vi "Autonomous Independent.vi"   [LabVIEW 2017]
doc: "This VI is called when autonomous begins, and will automatically be terminated when autonomous ends. You can carry out timed or sensor driven robot movement independently without needing to return to the caller."
uses:
  <vilib>/Rock Robotics/WPI/Utilities/WPI_GetSetVariantRefNum.vi
  <vilib>/Rock Robotics/Network Tables/NT Read String.vi
  <vilib>/Rock Robotics/Network Tables/NT Write Numeric Array.vi
panel:
  # "Be sure to right-click and choose Data Operations>>Make Current Value default if you want to save the array values with the VI"
types:
  T1 = typedef "WPI_JoystickDevRef.ctl" = cluster{"Device":T2}
  T2 = typedef "WPI_JoystickDeviceEnum.ctl" = enum16{"USB 0", "USB 1", "USB 2", "USB 3", "USB 4", "USB 5"}
  T3 = typedef "WPI_RobotDriveDevRef.ctl" = cluster{"DevStatus":errorcluster, "Motors[]":T4[], "Square Inputs":bool, "Max Output":dbl}
  T4 = typedef "WPI_MotorControlDeviceRef.ctl" = cluster{"DeviceStatus":errorcluster, "Type":T5, "PWM":cluster{"PWM Channel":T6, "DeadBand":T7}, "CAN":cluster{"Device Number":u8, "SetOutput VI Ref":variant, "GetOutput VI Ref":variant, "Enable VI Ref":variant, "Disable VI Ref":variant, "Data":variant}, "Invert":bool, "DIO PWM":cluster{"PWM \"Enable\" Channel":T6, "DIOChannel":T8, "PWM Rate":dbl}}
  T5 = typedef "WPI_MotorControlType.ctl" = enum16{"PWM", "CAN", "DIO PWM"}
  T6 = typedef "FPGA_DIOPWMChannel.ctl" = enum8{"PWM 0", "PWM 1", "PWM 2", "PWM 3", "PWM 4", "PWM 5", "PWM 6", "PWM 7", "PWM 8", "PWM 9", "PWM MXP 0", "PWM MXP 1", "PWM MXP 2", "PWM MXP 3", "PWM MXP 4", "PWM MXP 5", "PWM MXP 6", "PWM MXP 7", "PWM MXP 8", "PWM MXP 9", "Invalid"}
  T7 = typedef "WPI_PWMDeadband.ctl" = cluster{"Name":string, "maxPositivePwm":i32, "minPositivePwm":i32, "centerPwm":i32, "maxNegativePwm":i32, "minNegativePwm":i32, "angularRange":u16}
  T8 = typedef "FPGA_DIOChannel.ctl" = enum8{"DIO 0", "DIO 1", "DIO 2", "DIO 3", "DIO 4", "DIO 5", "DIO 6", "DIO 7", "DIO 8", "DIO 9", "DIO MXP 0", "DIO MXP 1", "DIO MXP 2", "DIO MXP 3", "DIO MXP 4", "DIO MXP 5", "DIO MXP 6", "DIO MXP 7", "DIO MXP 8", "DIO MXP 9", "DIO MXP 10", "DIO MXP 11", "DIO MXP 12", "DIO MXP 13", "DIO MXP 14", "DIO MXP 15", "SPI Port CS1", "SPI Port CS2", "SPI Port CS3", "SPI Port MISO", "SPI Port MOSI", "Invalid"}
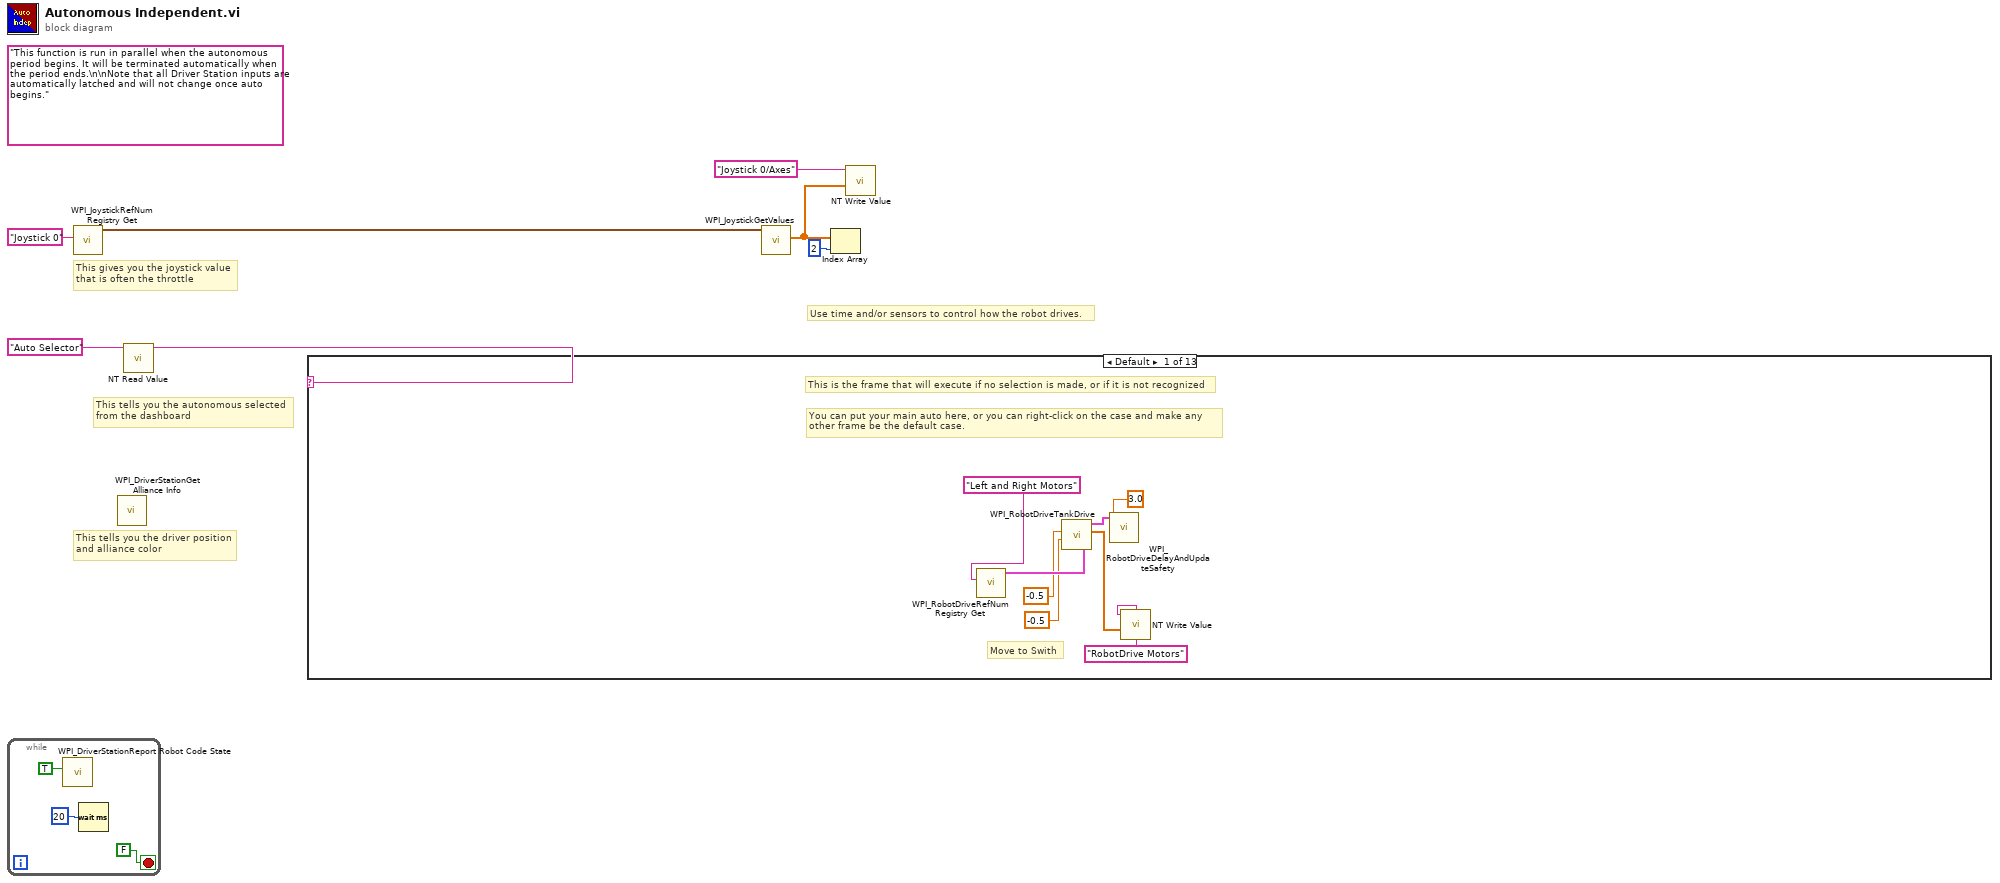
[diagram p0: block diagram]
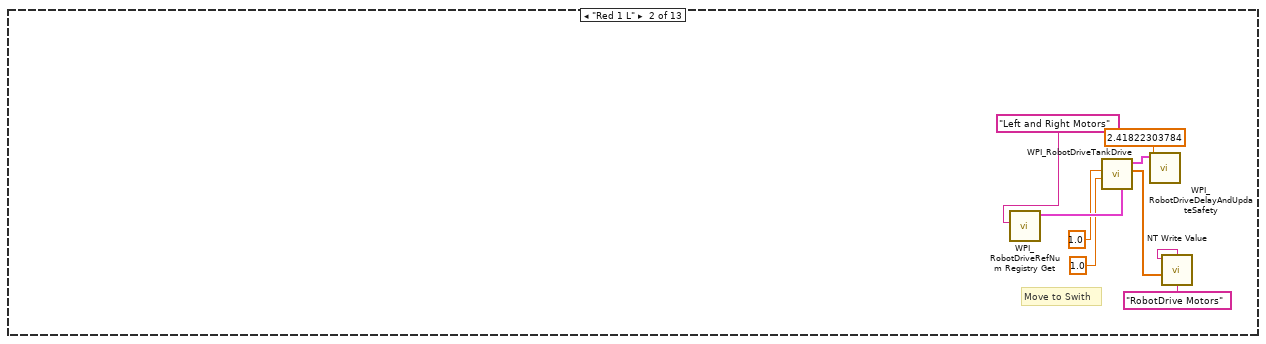
[diagram p2: hidden frame]
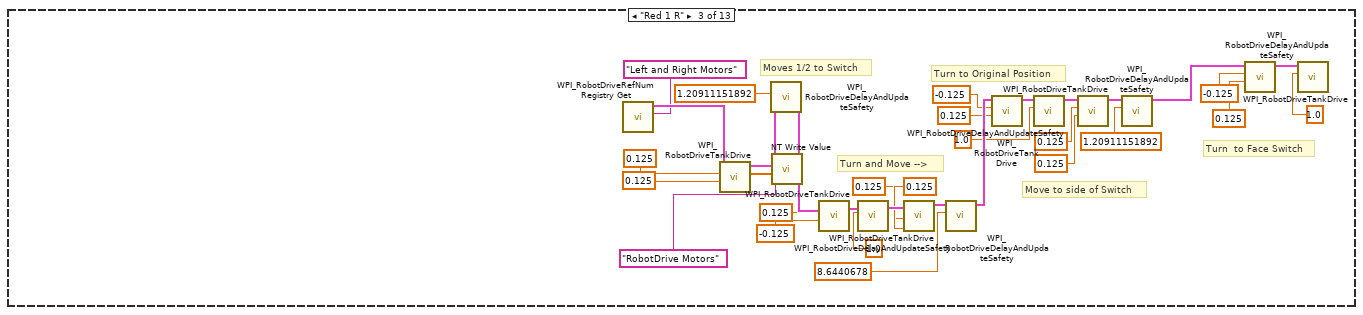
[diagram p3: hidden frame]
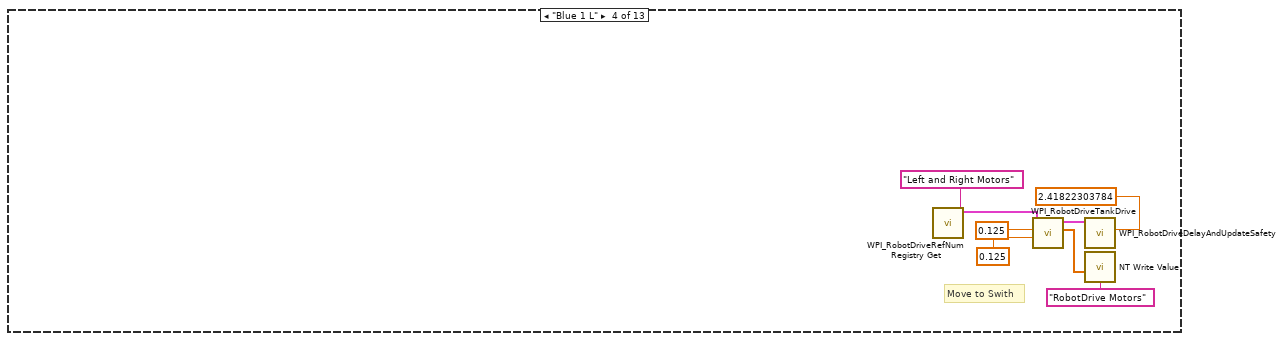
[diagram p4: hidden frame]
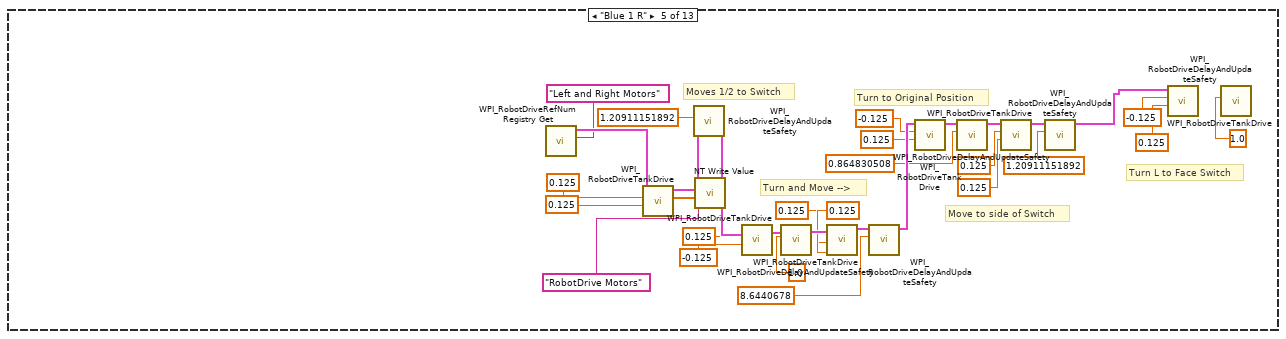
[diagram p5: hidden frame]
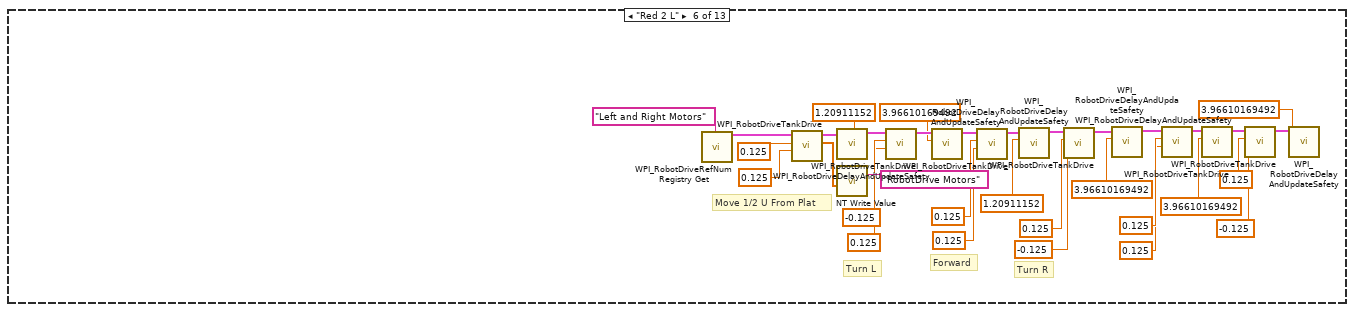
[diagram p6: hidden frame]
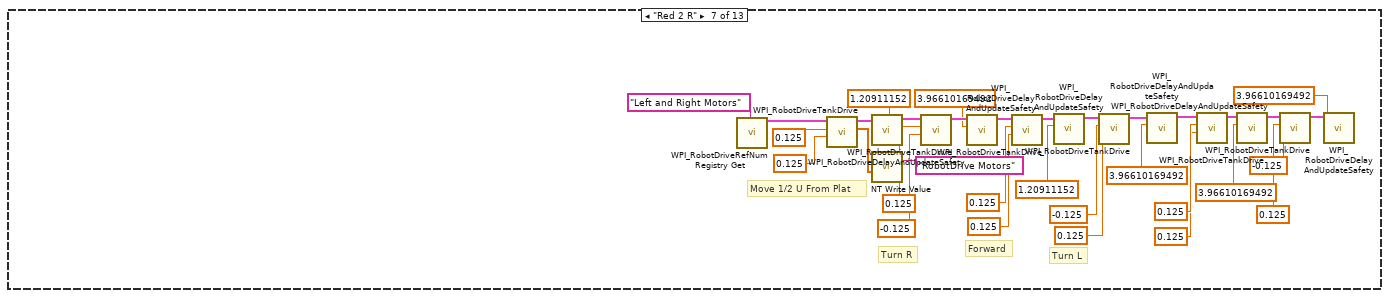
[diagram p7: hidden frame]
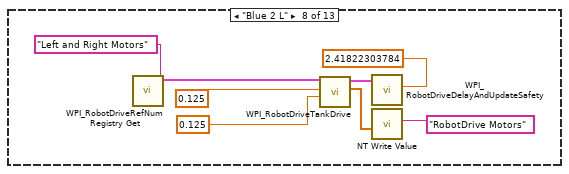
[diagram p8: hidden frame]
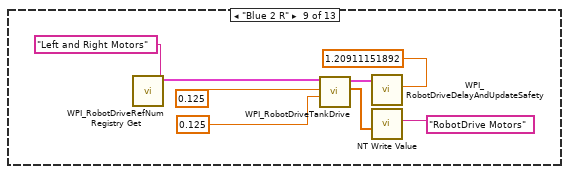
[diagram p9: hidden frame]
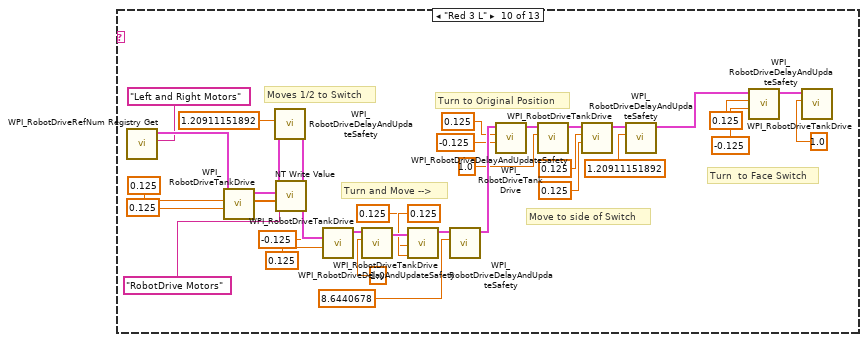
[diagram p10: hidden frame]
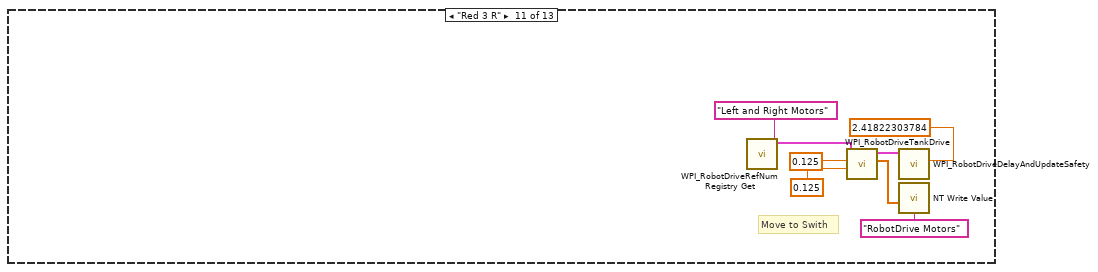
[diagram p11: hidden frame]
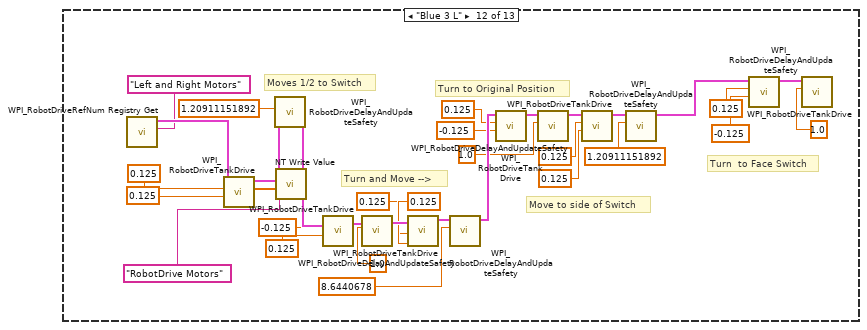
[diagram p12: hidden frame]
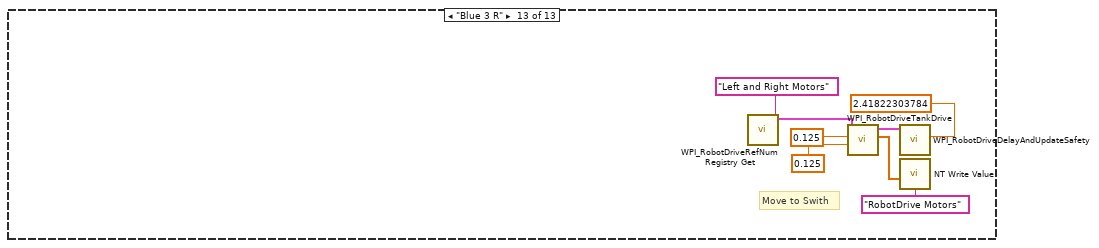
[diagram p13: hidden frame]
diagram:
  (unwired) "This function is run in parallel when the autonomous period begins. It will be terminated automatically when the period ends.\n\nNote that all Driver Station inputs are automatically latched and will not change once auto begins."
  # "This tells you the autonomous selected\nfrom the dashboard"
  # "This gives you the joystick value\nthat is often the throttle"
  # "Use time and/or sensors to control how the robot drives."
  # "This tells you the driver position\nand alliance color"
  n1 = while {
    stop <- FALSE stop-if-true
    n2 = call <vilib>:"WPI_DriverStationReport Robot Code State.vi"("Autonomous"=TRUE) -> ()  [unwired: 10 in, 1 out]
    n3 = Wait (ms)(milliseconds to wait=u32 20) -> ()  [unwired: 1 out]
  }
  n4 = call <vilib>:"WPI_JoystickRefNum Registry Get.vi"("refnum name"="Joystick 0") -> ("JoystickDevRef"=w6:T1)  [unwired: 1 in, 9 out]
  n5 = call <vilib>:"WPI_DriverStationGet Alliance Info.vi"() -> ()  [unwired: 12 out]
  n6 = call-poly <vilib>:"NT Read Value.vi"("Name"="Auto Selector") -> ("String"=w3:string)  [unwired: 9 in, 1 out]
  n7 = case shown="Default" w3 {
    frame Default {
      # "Move to Swith"
      # "You can put your main auto here, or you can right-click on the case and make any\nother frame be the default case."
      # "This is the frame that will execute if no selection is made, or if it is not recognized"
      n8 = call <vilib>:"WPI_RobotDriveRefNum Registry Get.vi"("refnum name"="Left and Right Motors") -> ("RobotDriveDevRef"=w16:T3)  [unwired: 1 in, 9 out]
      n9 = call <vilib>:"WPI_RobotDriveTankDrive.vi"("Right axis value"=-0.5 ("X axis value"), "Left axis value"=-0.5 ("X axis value"), "RobotDriveDevRef"=w16) -> ("Motor Values"=w18:dbl[], "RobotDriveDevRef"=w17:T3)  [unwired: 6 in, 1 out]
      n10 = call <vilib>:"WPI_RobotDriveDelayAndUpdateSafety.vi"("Delay (s)"=3.0, "RobotDriveDevRef"=w17) -> ()  [unwired: 8 in, 2 out]
      n11 = call-poly <vilib>:"NT Write Value.vi"("Numeric Array"=w18, "Name"="RobotDrive Motors") -> ()  [unwired: 9 in, 1 out]
    }
    frame "Red 1 L" {
      # "Move to Swith"
      n12 = call <vilib>:"WPI_RobotDriveRefNum Registry Get.vi"("refnum name"="Left and Right Motors") -> ("RobotDriveDevRef"=w24:T3)  [unwired: 1 in, 9 out]
      n13 = call <vilib>:"WPI_RobotDriveTankDrive.vi"("Right axis value"=1.0 ("X axis value"), "Left axis value"=1.0 ("X axis value"), "RobotDriveDevRef"=w24) -> ("Motor Values"=w26:dbl[], "RobotDriveDevRef"=w25:T3)  [unwired: 6 in, 1 out]
      n14 = call <vilib>:"WPI_RobotDriveDelayAndUpdateSafety.vi"("Delay (s)"=2.41822303784, "RobotDriveDevRef"=w25) -> ()  [unwired: 8 in, 2 out]
      n15 = call-poly <vilib>:"NT Write Value.vi"("Numeric Array"=w26, "Name"="RobotDrive Motors") -> ()  [unwired: 9 in, 1 out]
    }
    frame "Red 1 R" {
      # "Turn  to Face Switch"
      # "Move to side of Switch"
      # "Turn to Original Position"
      # "Turn and Move -->"
      # "Moves 1/2 to Switch"
      n16 = call <vilib>:"WPI_RobotDriveRefNum Registry Get.vi"("refnum name"="Left and Right Motors") -> ("RobotDriveDevRef"=w59:T3)  [unwired: 1 in, 9 out]
      n17 = call <vilib>:"WPI_RobotDriveTankDrive.vi"("Right axis value"=0.125 ("X axis value"), "Left axis value"=0.125 ("X axis value"), "RobotDriveDevRef"=w59) -> ("Motor Values"=w54:dbl[], "RobotDriveDevRef"=w56:T3)  [unwired: 6 in, 1 out]
      n18 = call <vilib>:"WPI_RobotDriveDelayAndUpdateSafety.vi"("Delay (s)"=1.20911151892, "RobotDriveDevRef"=w56) -> ("RobotDriveDevRef 2"=w52:T3)  [unwired: 8 in, 1 out]
      n19 = call-poly <vilib>:"NT Write Value.vi"("Numeric Array"=w54, "Name"="RobotDrive Motors") -> ()  [unwired: 9 in, 1 out]
      n20 = call <vilib>:"WPI_RobotDriveTankDrive.vi"("Right axis value"=-0.125, "Left axis value"=0.125, "RobotDriveDevRef"=w52) -> ("RobotDriveDevRef"=w48:T3)  [unwired: 6 in, 2 out]
      n21 = call <vilib>:"WPI_RobotDriveDelayAndUpdateSafety.vi"("Delay (s)"=1.0, "RobotDriveDevRef"=w48) -> ("RobotDriveDevRef 2"=w46:T3)  [unwired: 8 in, 1 out]
      n22 = call <vilib>:"WPI_RobotDriveTankDrive.vi"("Right axis value"=0.125, "Left axis value"=0.125, "RobotDriveDevRef"=w46) -> ("RobotDriveDevRef"=w45:T3)  [unwired: 6 in, 2 out]
      n23 = call <vilib>:"WPI_RobotDriveDelayAndUpdateSafety.vi"("Delay (s)"=8.6440678, "RobotDriveDevRef"=w45) -> ("RobotDriveDevRef 2"=w41:T3)  [unwired: 8 in, 1 out]
      n24 = call <vilib>:"WPI_RobotDriveTankDrive.vi"("Right axis value"=0.125, "Left axis value"=-0.125, "RobotDriveDevRef"=w41) -> ("RobotDriveDevRef"=w38:T3)  [unwired: 6 in, 2 out]
      n25 = call <vilib>:"WPI_RobotDriveDelayAndUpdateSafety.vi"("Delay (s)"=1.0, "RobotDriveDevRef"=w38) -> ("RobotDriveDevRef 2"=w36:T3)  [unwired: 8 in, 1 out]
      n26 = call <vilib>:"WPI_RobotDriveTankDrive.vi"("Right axis value"=0.125, "Left axis value"=0.125, "RobotDriveDevRef"=w36) -> ("RobotDriveDevRef"=w33:T3)  [unwired: 6 in, 2 out]
      n27 = call <vilib>:"WPI_RobotDriveDelayAndUpdateSafety.vi"("Delay (s)"=1.20911151892, "RobotDriveDevRef"=w33) -> ("RobotDriveDevRef 2"=w31:T3)  [unwired: 8 in, 1 out]
      n28 = call <vilib>:"WPI_RobotDriveTankDrive.vi"("Right axis value"=0.125, "Left axis value"=-0.125, "RobotDriveDevRef"=w31) -> ("RobotDriveDevRef"=w28:T3)  [unwired: 6 in, 2 out]
      n29 = call <vilib>:"WPI_RobotDriveDelayAndUpdateSafety.vi"("Delay (s)"=1.0, "RobotDriveDevRef"=w28) -> ()  [unwired: 8 in, 2 out]
    }
    frame "Blue 1 L" {
      # "Move to Swith"
      n30 = call <vilib>:"WPI_RobotDriveRefNum Registry Get.vi"("refnum name"="Left and Right Motors") -> ("RobotDriveDevRef"=w67:T3)  [unwired: 1 in, 9 out]
      n31 = call <vilib>:"WPI_RobotDriveTankDrive.vi"("Right axis value"=0.125 ("X axis value"), "Left axis value"=0.125 ("X axis value"), "RobotDriveDevRef"=w67) -> ("Motor Values"=w62:dbl[], "RobotDriveDevRef"=w64:T3)  [unwired: 6 in, 1 out]
      n32 = call <vilib>:"WPI_RobotDriveDelayAndUpdateSafety.vi"("Delay (s)"=2.41822303784, "RobotDriveDevRef"=w64) -> ()  [unwired: 8 in, 2 out]
      n33 = call-poly <vilib>:"NT Write Value.vi"("Numeric Array"=w62, "Name"="RobotDrive Motors") -> ()  [unwired: 9 in, 1 out]
    }
    frame "Blue 1 R" {
      # "Turn L to Face Switch"
      # "Move to side of Switch"
      # "Turn to Original Position"
      # "Turn and Move -->"
      # "Moves 1/2 to Switch"
      n34 = call <vilib>:"WPI_RobotDriveRefNum Registry Get.vi"("refnum name"="Left and Right Motors") -> ("RobotDriveDevRef"=w99:T3)  [unwired: 1 in, 9 out]
      n35 = call <vilib>:"WPI_RobotDriveTankDrive.vi"("Right axis value"=0.125 ("X axis value"), "Left axis value"=0.125 ("X axis value"), "RobotDriveDevRef"=w99) -> ("Motor Values"=w94:dbl[], "RobotDriveDevRef"=w96:T3)  [unwired: 6 in, 1 out]
      n36 = call <vilib>:"WPI_RobotDriveDelayAndUpdateSafety.vi"("Delay (s)"=1.20911151892, "RobotDriveDevRef"=w96) -> ("RobotDriveDevRef 2"=w92:T3)  [unwired: 8 in, 1 out]
      n37 = call-poly <vilib>:"NT Write Value.vi"("Numeric Array"=w94, "Name"="RobotDrive Motors") -> ()  [unwired: 9 in, 1 out]
      n38 = call <vilib>:"WPI_RobotDriveTankDrive.vi"("Right axis value"=-0.125, "Left axis value"=0.125, "RobotDriveDevRef"=w92) -> ("RobotDriveDevRef"=w88:T3)  [unwired: 6 in, 2 out]
      n39 = call <vilib>:"WPI_RobotDriveDelayAndUpdateSafety.vi"("Delay (s)"=1.0, "RobotDriveDevRef"=w88) -> ("RobotDriveDevRef 2"=w86:T3)  [unwired: 8 in, 1 out]
      n40 = call <vilib>:"WPI_RobotDriveTankDrive.vi"("Right axis value"=0.125, "Left axis value"=0.125, "RobotDriveDevRef"=w86) -> ("RobotDriveDevRef"=w85:T3)  [unwired: 6 in, 2 out]
      n41 = call <vilib>:"WPI_RobotDriveDelayAndUpdateSafety.vi"("Delay (s)"=8.6440678, "RobotDriveDevRef"=w85) -> ("RobotDriveDevRef 2"=w81:T3)  [unwired: 8 in, 1 out]
      n42 = call <vilib>:"WPI_RobotDriveTankDrive.vi"("Right axis value"=0.125, "Left axis value"=-0.125, "RobotDriveDevRef"=w81) -> ("RobotDriveDevRef"=w78:T3)  [unwired: 6 in, 2 out]
      n43 = call <vilib>:"WPI_RobotDriveDelayAndUpdateSafety.vi"("Delay (s)"=0.864830508, "RobotDriveDevRef"=w78) -> ("RobotDriveDevRef 2"=w76:T3)  [unwired: 8 in, 1 out]
      n44 = call <vilib>:"WPI_RobotDriveTankDrive.vi"("Right axis value"=0.125, "Left axis value"=0.125, "RobotDriveDevRef"=w76) -> ("RobotDriveDevRef"=w73:T3)  [unwired: 6 in, 2 out]
      n45 = call <vilib>:"WPI_RobotDriveDelayAndUpdateSafety.vi"("Delay (s)"=1.20911151892, "RobotDriveDevRef"=w73) -> ("RobotDriveDevRef 2"=w68:T3)  [unwired: 8 in, 1 out]
      n46 = call <vilib>:"WPI_RobotDriveTankDrive.vi"("Right axis value"=0.125, "Left axis value"=-0.125, "RobotDriveDevRef"=w68) -> ()  [unwired: 6 in, 3 out]
      n47 = call <vilib>:"WPI_RobotDriveDelayAndUpdateSafety.vi"("Delay (s)"=1.0) -> ()  [unwired: 9 in, 2 out]
    }
    frame "Red 2 L" {
      # "Forward"
      # "Turn R"
      # "Turn L"
      # "Move 1/2 U From Plat"
      n48 = call <vilib>:"WPI_RobotDriveRefNum Registry Get.vi"("refnum name"="Left and Right Motors") -> ("RobotDriveDevRef"=w132:T3)  [unwired: 1 in, 9 out]
      n49 = call <vilib>:"WPI_RobotDriveTankDrive.vi"("Right axis value"=0.125 ("X axis value"), "Left axis value"=0.125 ("X axis value"), "RobotDriveDevRef"=w132) -> ("Motor Values"=w127:dbl[], "RobotDriveDevRef"=w129:T3)  [unwired: 6 in, 1 out]
      n50 = call <vilib>:"WPI_RobotDriveDelayAndUpdateSafety.vi"("Delay (s)"=1.20911152, "RobotDriveDevRef"=w129) -> ("RobotDriveDevRef 2"=w124:T3)  [unwired: 8 in, 1 out]
      n51 = call-poly <vilib>:"NT Write Value.vi"("Numeric Array"=w127, "Name"="RobotDrive Motors") -> ()  [unwired: 9 in, 1 out]
      n52 = call <vilib>:"WPI_RobotDriveTankDrive.vi"("Right axis value"=0.125, "Left axis value"=-0.125, "RobotDriveDevRef"=w124) -> ("RobotDriveDevRef"=w121:T3)  [unwired: 6 in, 2 out]
      n53 = call <vilib>:"WPI_RobotDriveDelayAndUpdateSafety.vi"("Delay (s)"=3.96610169492, "RobotDriveDevRef"=w121) -> ("RobotDriveDevRef 2"=w119:T3)  [unwired: 8 in, 1 out]
      n54 = call <vilib>:"WPI_RobotDriveTankDrive.vi"("Right axis value"=0.125, "Left axis value"=0.125, "RobotDriveDevRef"=w119) -> ("RobotDriveDevRef"=w116:T3)  [unwired: 6 in, 2 out]
      n55 = call <vilib>:"WPI_RobotDriveDelayAndUpdateSafety.vi"("Delay (s)"=1.20911152, "RobotDriveDevRef"=w116) -> ("RobotDriveDevRef 2"=w114:T3)  [unwired: 8 in, 1 out]
      n56 = call <vilib>:"WPI_RobotDriveTankDrive.vi"("Right axis value"=-0.125, "Left axis value"=0.125, "RobotDriveDevRef"=w114) -> ("RobotDriveDevRef"=w112:T3)  [unwired: 6 in, 2 out]
      n57 = call <vilib>:"WPI_RobotDriveDelayAndUpdateSafety.vi"("Delay (s)"=3.96610169492, "RobotDriveDevRef"=w112) -> ("RobotDriveDevRef 2"=w109:T3)  [unwired: 8 in, 1 out]
      n58 = call <vilib>:"WPI_RobotDriveTankDrive.vi"("Right axis value"=0.125, "Left axis value"=0.125, "RobotDriveDevRef"=w109) -> ("RobotDriveDevRef"=w106:T3)  [unwired: 6 in, 2 out]
      n59 = call <vilib>:"WPI_RobotDriveDelayAndUpdateSafety.vi"("Delay (s)"=3.96610169492, "RobotDriveDevRef"=w106) -> ("RobotDriveDevRef 2"=w104:T3)  [unwired: 8 in, 1 out]
      n60 = call <vilib>:"WPI_RobotDriveTankDrive.vi"("Right axis value"=-0.125, "Left axis value"=0.125, "RobotDriveDevRef"=w104) -> ("RobotDriveDevRef"=w101:T3)  [unwired: 6 in, 2 out]
      n61 = call <vilib>:"WPI_RobotDriveDelayAndUpdateSafety.vi"("Delay (s)"=3.96610169492, "RobotDriveDevRef"=w101) -> ()  [unwired: 8 in, 2 out]
    }
    frame "Red 2 R" {
      # "Forward"
      # "Turn L"
      # "Turn R"
      # "Move 1/2 U From Plat"
      n62 = call <vilib>:"WPI_RobotDriveRefNum Registry Get.vi"("refnum name"="Left and Right Motors") -> ("RobotDriveDevRef"=w165:T3)  [unwired: 1 in, 9 out]
      n63 = call <vilib>:"WPI_RobotDriveTankDrive.vi"("Right axis value"=0.125 ("X axis value"), "Left axis value"=0.125 ("X axis value"), "RobotDriveDevRef"=w165) -> ("Motor Values"=w160:dbl[], "RobotDriveDevRef"=w162:T3)  [unwired: 6 in, 1 out]
      n64 = call <vilib>:"WPI_RobotDriveDelayAndUpdateSafety.vi"("Delay (s)"=1.20911152, "RobotDriveDevRef"=w162) -> ("RobotDriveDevRef 2"=w157:T3)  [unwired: 8 in, 1 out]
      n65 = call-poly <vilib>:"NT Write Value.vi"("Numeric Array"=w160, "Name"="RobotDrive Motors") -> ()  [unwired: 9 in, 1 out]
      n66 = call <vilib>:"WPI_RobotDriveTankDrive.vi"("Right axis value"=-0.125, "Left axis value"=0.125, "RobotDriveDevRef"=w157) -> ("RobotDriveDevRef"=w154:T3)  [unwired: 6 in, 2 out]
      n67 = call <vilib>:"WPI_RobotDriveDelayAndUpdateSafety.vi"("Delay (s)"=3.96610169492, "RobotDriveDevRef"=w154) -> ("RobotDriveDevRef 2"=w152:T3)  [unwired: 8 in, 1 out]
      n68 = call <vilib>:"WPI_RobotDriveTankDrive.vi"("Right axis value"=0.125, "Left axis value"=0.125, "RobotDriveDevRef"=w152) -> ("RobotDriveDevRef"=w149:T3)  [unwired: 6 in, 2 out]
      n69 = call <vilib>:"WPI_RobotDriveDelayAndUpdateSafety.vi"("Delay (s)"=1.20911152, "RobotDriveDevRef"=w149) -> ("RobotDriveDevRef 2"=w147:T3)  [unwired: 8 in, 1 out]
      n70 = call <vilib>:"WPI_RobotDriveTankDrive.vi"("Right axis value"=0.125, "Left axis value"=-0.125, "RobotDriveDevRef"=w147) -> ("RobotDriveDevRef"=w145:T3)  [unwired: 6 in, 2 out]
      n71 = call <vilib>:"WPI_RobotDriveDelayAndUpdateSafety.vi"("Delay (s)"=3.96610169492, "RobotDriveDevRef"=w145) -> ("RobotDriveDevRef 2"=w142:T3)  [unwired: 8 in, 1 out]
      n72 = call <vilib>:"WPI_RobotDriveTankDrive.vi"("Right axis value"=0.125, "Left axis value"=0.125, "RobotDriveDevRef"=w142) -> ("RobotDriveDevRef"=w139:T3)  [unwired: 6 in, 2 out]
      n73 = call <vilib>:"WPI_RobotDriveDelayAndUpdateSafety.vi"("Delay (s)"=3.96610169492, "RobotDriveDevRef"=w139) -> ("RobotDriveDevRef 2"=w137:T3)  [unwired: 8 in, 1 out]
      n74 = call <vilib>:"WPI_RobotDriveTankDrive.vi"("Right axis value"=0.125, "Left axis value"=-0.125, "RobotDriveDevRef"=w137) -> ("RobotDriveDevRef"=w134:T3)  [unwired: 6 in, 2 out]
      n75 = call <vilib>:"WPI_RobotDriveDelayAndUpdateSafety.vi"("Delay (s)"=3.96610169492, "RobotDriveDevRef"=w134) -> ()  [unwired: 8 in, 2 out]
    }
    frame "Blue 2 L" {
      n76 = call <vilib>:"WPI_RobotDriveRefNum Registry Get.vi"("refnum name"="Left and Right Motors") -> ("RobotDriveDevRef"=w173:T3)  [unwired: 1 in, 9 out]
      n77 = call <vilib>:"WPI_RobotDriveTankDrive.vi"("Right axis value"=0.125 ("X axis value"), "Left axis value"=0.125 ("X axis value"), "RobotDriveDevRef"=w173) -> ("Motor Values"=w168:dbl[], "RobotDriveDevRef"=w170:T3)  [unwired: 6 in, 1 out]
      n78 = call <vilib>:"WPI_RobotDriveDelayAndUpdateSafety.vi"("Delay (s)"=2.41822303784, "RobotDriveDevRef"=w170) -> ()  [unwired: 8 in, 2 out]
      n79 = call-poly <vilib>:"NT Write Value.vi"("Numeric Array"=w168, "Name"="RobotDrive Motors") -> ()  [unwired: 9 in, 1 out]
    }
    frame "Blue 2 R" {
      n80 = call <vilib>:"WPI_RobotDriveRefNum Registry Get.vi"("refnum name"="Left and Right Motors") -> ("RobotDriveDevRef"=w181:T3)  [unwired: 1 in, 9 out]
      n81 = call <vilib>:"WPI_RobotDriveTankDrive.vi"("Right axis value"=0.125 ("X axis value"), "Left axis value"=0.125 ("X axis value"), "RobotDriveDevRef"=w181) -> ("Motor Values"=w176:dbl[], "RobotDriveDevRef"=w178:T3)  [unwired: 6 in, 1 out]
      n82 = call <vilib>:"WPI_RobotDriveDelayAndUpdateSafety.vi"("Delay (s)"=1.20911151892, "RobotDriveDevRef"=w178) -> ()  [unwired: 8 in, 2 out]
      n83 = call-poly <vilib>:"NT Write Value.vi"("Numeric Array"=w176, "Name"="RobotDrive Motors") -> ()  [unwired: 9 in, 1 out]
    }
    frame "Red 3 L" {
      # "Turn  to Face Switch"
      # "Move to side of Switch"
      # "Turn to Original Position"
      # "Turn and Move -->"
      # "Moves 1/2 to Switch"
      n84 = call <vilib>:"WPI_RobotDriveRefNum Registry Get.vi"("refnum name"="Left and Right Motors") -> ("RobotDriveDevRef"=w214:T3)  [unwired: 1 in, 9 out]
      n85 = call <vilib>:"WPI_RobotDriveTankDrive.vi"("Right axis value"=0.125 ("X axis value"), "Left axis value"=0.125 ("X axis value"), "RobotDriveDevRef"=w214) -> ("Motor Values"=w209:dbl[], "RobotDriveDevRef"=w211:T3)  [unwired: 6 in, 1 out]
      n86 = call <vilib>:"WPI_RobotDriveDelayAndUpdateSafety.vi"("Delay (s)"=1.20911151892, "RobotDriveDevRef"=w211) -> ("RobotDriveDevRef 2"=w207:T3)  [unwired: 8 in, 1 out]
      n87 = call-poly <vilib>:"NT Write Value.vi"("Numeric Array"=w209, "Name"="RobotDrive Motors") -> ()  [unwired: 9 in, 1 out]
      n88 = call <vilib>:"WPI_RobotDriveTankDrive.vi"("Right axis value"=0.125, "Left axis value"=-0.125, "RobotDriveDevRef"=w207) -> ("RobotDriveDevRef"=w182:T3)  [unwired: 6 in, 2 out]
      n89 = call <vilib>:"WPI_RobotDriveDelayAndUpdateSafety.vi"("Delay (s)"=1.0, "RobotDriveDevRef"=w182) -> ("RobotDriveDevRef 2"=w202:T3)  [unwired: 8 in, 1 out]
      n90 = call <vilib>:"WPI_RobotDriveTankDrive.vi"("Right axis value"=0.125, "Left axis value"=0.125, "RobotDriveDevRef"=w202) -> ("RobotDriveDevRef"=w201:T3)  [unwired: 6 in, 2 out]
      n91 = call <vilib>:"WPI_RobotDriveDelayAndUpdateSafety.vi"("Delay (s)"=8.6440678, "RobotDriveDevRef"=w201) -> ("RobotDriveDevRef 2"=w197:T3)  [unwired: 8 in, 1 out]
      n92 = call <vilib>:"WPI_RobotDriveTankDrive.vi"("Right axis value"=-0.125, "Left axis value"=0.125, "RobotDriveDevRef"=w197) -> ("RobotDriveDevRef"=w194:T3)  [unwired: 6 in, 2 out]
      n93 = call <vilib>:"WPI_RobotDriveDelayAndUpdateSafety.vi"("Delay (s)"=1.0, "RobotDriveDevRef"=w194) -> ("RobotDriveDevRef 2"=w192:T3)  [unwired: 8 in, 1 out]
      n94 = call <vilib>:"WPI_RobotDriveTankDrive.vi"("Right axis value"=0.125, "Left axis value"=0.125, "RobotDriveDevRef"=w192) -> ("RobotDriveDevRef"=w189:T3)  [unwired: 6 in, 2 out]
      n95 = call <vilib>:"WPI_RobotDriveDelayAndUpdateSafety.vi"("Delay (s)"=1.20911151892, "RobotDriveDevRef"=w189) -> ("RobotDriveDevRef 2"=w187:T3)  [unwired: 8 in, 1 out]
      n96 = call <vilib>:"WPI_RobotDriveTankDrive.vi"("Right axis value"=-0.125, "Left axis value"=0.125, "RobotDriveDevRef"=w187) -> ("RobotDriveDevRef"=w184:T3)  [unwired: 6 in, 2 out]
      n97 = call <vilib>:"WPI_RobotDriveDelayAndUpdateSafety.vi"("Delay (s)"=1.0, "RobotDriveDevRef"=w184) -> ()  [unwired: 8 in, 2 out]
    }
    frame "Red 3 R" {
      # "Move to Swith"
      n98 = call <vilib>:"WPI_RobotDriveRefNum Registry Get.vi"("refnum name"="Left and Right Motors") -> ("RobotDriveDevRef"=w222:T3)  [unwired: 1 in, 9 out]
      n99 = call <vilib>:"WPI_RobotDriveTankDrive.vi"("Right axis value"=0.125 ("X axis value"), "Left axis value"=0.125 ("X axis value"), "RobotDriveDevRef"=w222) -> ("Motor Values"=w218:dbl[], "RobotDriveDevRef"=w220:T3)  [unwired: 6 in, 1 out]
      n100 = call <vilib>:"WPI_RobotDriveDelayAndUpdateSafety.vi"("Delay (s)"=2.41822303784, "RobotDriveDevRef"=w220) -> ()  [unwired: 8 in, 2 out]
      n101 = call-poly <vilib>:"NT Write Value.vi"("Numeric Array"=w218, "Name"="RobotDrive Motors") -> ()  [unwired: 9 in, 1 out]
    }
    frame "Blue 3 L" {
      # "Turn  to Face Switch"
      # "Move to side of Switch"
      # "Turn to Original Position"
      # "Turn and Move -->"
      # "Moves 1/2 to Switch"
      n102 = call <vilib>:"WPI_RobotDriveRefNum Registry Get.vi"("refnum name"="Left and Right Motors") -> ("RobotDriveDevRef"=w255:T3)  [unwired: 1 in, 9 out]
      n103 = call <vilib>:"WPI_RobotDriveTankDrive.vi"("Right axis value"=0.125 ("X axis value"), "Left axis value"=0.125 ("X axis value"), "RobotDriveDevRef"=w255) -> ("Motor Values"=w250:dbl[], "RobotDriveDevRef"=w252:T3)  [unwired: 6 in, 1 out]
      n104 = call <vilib>:"WPI_RobotDriveDelayAndUpdateSafety.vi"("Delay (s)"=1.20911151892, "RobotDriveDevRef"=w252) -> ("RobotDriveDevRef 2"=w248:T3)  [unwired: 8 in, 1 out]
      n105 = call-poly <vilib>:"NT Write Value.vi"("Numeric Array"=w250, "Name"="RobotDrive Motors") -> ()  [unwired: 9 in, 1 out]
      n106 = call <vilib>:"WPI_RobotDriveTankDrive.vi"("Right axis value"=0.125, "Left axis value"=-0.125, "RobotDriveDevRef"=w248) -> ("RobotDriveDevRef"=w244:T3)  [unwired: 6 in, 2 out]
      n107 = call <vilib>:"WPI_RobotDriveDelayAndUpdateSafety.vi"("Delay (s)"=1.0, "RobotDriveDevRef"=w244) -> ("RobotDriveDevRef 2"=w242:T3)  [unwired: 8 in, 1 out]
      n108 = call <vilib>:"WPI_RobotDriveTankDrive.vi"("Right axis value"=0.125, "Left axis value"=0.125, "RobotDriveDevRef"=w242) -> ("RobotDriveDevRef"=w241:T3)  [unwired: 6 in, 2 out]
      n109 = call <vilib>:"WPI_RobotDriveDelayAndUpdateSafety.vi"("Delay (s)"=8.6440678, "RobotDriveDevRef"=w241) -> ("RobotDriveDevRef 2"=w237:T3)  [unwired: 8 in, 1 out]
      n110 = call <vilib>:"WPI_RobotDriveTankDrive.vi"("Right axis value"=-0.125, "Left axis value"=0.125, "RobotDriveDevRef"=w237) -> ("RobotDriveDevRef"=w234:T3)  [unwired: 6 in, 2 out]
      n111 = call <vilib>:"WPI_RobotDriveDelayAndUpdateSafety.vi"("Delay (s)"=1.0, "RobotDriveDevRef"=w234) -> ("RobotDriveDevRef 2"=w232:T3)  [unwired: 8 in, 1 out]
      n112 = call <vilib>:"WPI_RobotDriveTankDrive.vi"("Right axis value"=0.125, "Left axis value"=0.125, "RobotDriveDevRef"=w232) -> ("RobotDriveDevRef"=w229:T3)  [unwired: 6 in, 2 out]
      n113 = call <vilib>:"WPI_RobotDriveDelayAndUpdateSafety.vi"("Delay (s)"=1.20911151892, "RobotDriveDevRef"=w229) -> ("RobotDriveDevRef 2"=w223:T3)  [unwired: 8 in, 1 out]
      n114 = call <vilib>:"WPI_RobotDriveTankDrive.vi"("Right axis value"=-0.125, "Left axis value"=0.125, "RobotDriveDevRef"=w223) -> ("RobotDriveDevRef"=w225:T3)  [unwired: 6 in, 2 out]
      n115 = call <vilib>:"WPI_RobotDriveDelayAndUpdateSafety.vi"("Delay (s)"=1.0, "RobotDriveDevRef"=w225) -> ()  [unwired: 8 in, 2 out]
    }
    frame "Blue 3 R" {
      # "Move to Swith"
      n116 = call <vilib>:"WPI_RobotDriveRefNum Registry Get.vi"("refnum name"="Left and Right Motors") -> ("RobotDriveDevRef"=w263:T3)  [unwired: 1 in, 9 out]
      n117 = call <vilib>:"WPI_RobotDriveTankDrive.vi"("Right axis value"=0.125 ("X axis value"), "Left axis value"=0.125 ("X axis value"), "RobotDriveDevRef"=w263) -> ("Motor Values"=w259:dbl[], "RobotDriveDevRef"=w261:T3)  [unwired: 6 in, 1 out]
      n118 = call <vilib>:"WPI_RobotDriveDelayAndUpdateSafety.vi"("Delay (s)"=2.41822303784, "RobotDriveDevRef"=w261) -> ()  [unwired: 8 in, 2 out]
      n119 = call-poly <vilib>:"NT Write Value.vi"("Numeric Array"=w259, "Name"="RobotDrive Motors") -> ()  [unwired: 9 in, 1 out]
    }
  }
  n120 = call <vilib>:"WPI_JoystickGetValues.vi"("JoystickDevRef"=w6) -> ("Axes"=w2:dbl[])  [unwired: 6 in, 4 out]
  n121 = Index Array(array=w2, index=2) -> ()  [unwired: 1 out]
  n122 = call-poly <vilib>:"NT Write Value.vi"("Numeric Array"=w2, "Name"="Joystick 0/Axes") -> ()  [unwired: 9 in, 1 out]
